vi "center_particle.vi"(0 "input_xyz":T4, 5 "tolerance":dbl=1e-06 format="%#_13g", 7 "max_iterations":i32=10, 9 "parameters_xy-scan":T2={"image_size_xy_um"=1.0, "frame_size_xy_px"=10, "dwell_time_ms"=1.0} {"dwell_time_ms" format="%#_13g"; "image_size_xy_um" format="%#_13g"}, 11 "parameters_z-scan":T1={"dwell_time_ms"=10.0, "q_steps"=10, "span_um"=1.0, "refocus"=TRUE} {"dwell_time_ms" format="%#_13g"}, 12 "autocorrect":bool=TRUE) -> (4 "output_xyz":T3, 6 "mini_scan":dbl[][](array[numeric]), 8 "timestamp":timestamp, 15 "particle_lost":bool)   [LabVIEW 2018]
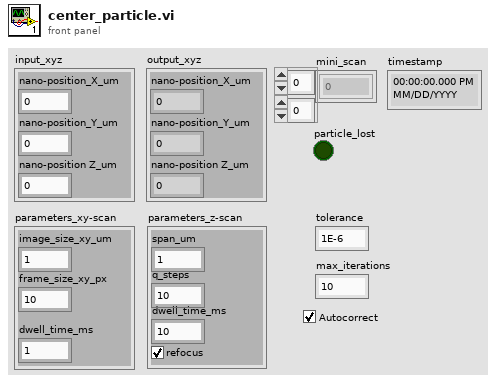
[diagram p1: front panel]
types:
  T1 = cluster{"dwell_time_ms":dbl, "q_steps":u32, "span_um":dbl, "refocus":bool}
  T2 = cluster{"image_size_xy_um":dbl, "frame_size_xy_px":u32, "dwell_time_ms":dbl}
  T3 = cluster{"nano-position_X_um":sgl, "nano-position_Y_um":sgl, "nano-position Z_um":sgl}
  T4 = cluster{"nano-position_X_um":dbl, "nano-position_Y_um":dbl, "nano-position Z_um":dbl}
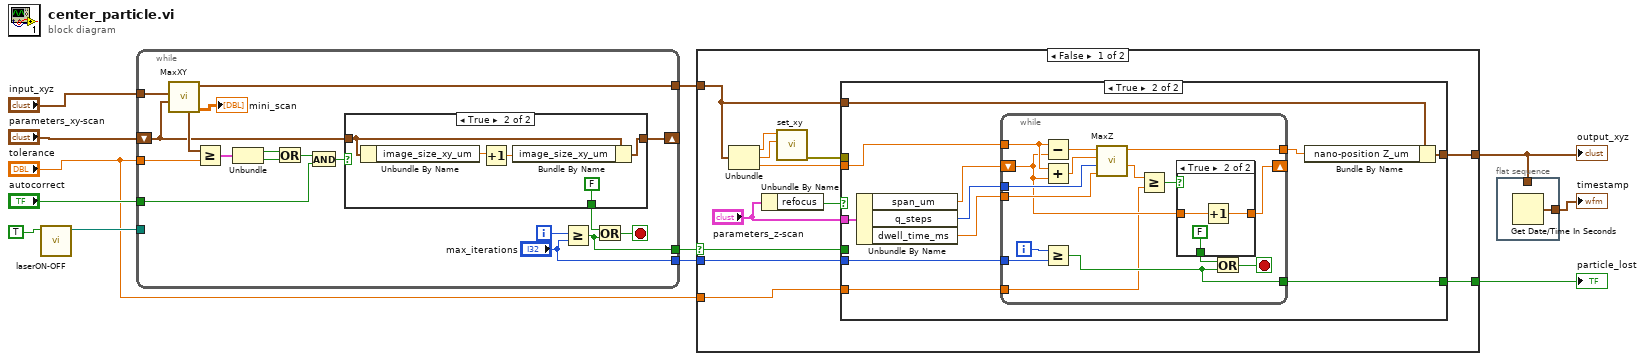
[diagram p0: block diagram]
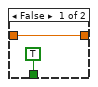
[diagram p3: hidden frame]
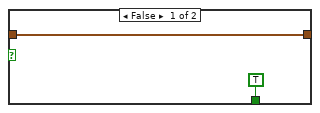
[diagram p5: hidden frame]
diagram:
  n1 = call "laserON-OFF.vi"("ON-OFF"=TRUE) -> ("path out"=w8:path)  [unwired: 10 in]
  n2 = while {
    tunnel: "input_xyz" -> [w30]
    tunnel: [w29] -> w11
    shift-right: [w22] -> _
    shift-left: "parameters_xy-scan" -> [w21]
    tunnel: "tolerance" -> [w16]
    tunnel: "autocorrect" -> [w15]
    tunnel: w8 -> [_]
    tunnel: [w14] -> w7
    tunnel: ["max_iterations"] -> w6
    i -> [w23]
    stop <- w20 stop-if-true
    n3 = call "MaxXY.vi"("input_xyz_um"=w30, "parameters_xy_scan"=w21) -> ("mse"=w27:cluster{"mse_y":dbl, "mse_x":dbl}, "output_xyz_um"=w29:T3, "image"=→"mini_scan":dbl[][])  [unwired: 4 in, 2 out]
    n4 = Greater Or Equal?(x=w27, y=w16) -> (x >= y?=w26:cluster{"mse_y":bool, "mse_x":bool})
    n5 = Unbundle(w26) -> ("mse_y"=w25:bool, "mse_x"=w24:bool)
    n6 = Or(x=w25, y=w24) -> (x .or. y?=w18:bool)
    n7 = And(x=w18, y=w15) -> (x .and. y?=w17:bool)
    n8 = case shown="True" w17 {
      tunnel: [w32 w33] -> w22
      tunnel: w21 -> [w32 w35]
      tunnel: [TRUE FALSE] -> w19
      frame False {
      }
      frame True {
        n9 = Unbundle By Name(w35) -> ("image_size_xy_um"=w36:dbl)
        n10 = Increment(x=w36) -> (x+1=w34:dbl)
        n11 = Bundle By Name(cluster=w35, "image_size_xy_um"=w34) -> (w33:T2)
      }
    }
    n12 = Greater Or Equal?(x=w23, y="max_iterations") -> (x >= y?=w14:bool)
    n13 = Or(x=w19, y=w14) -> (x .or. y?=w20:bool)
  }
  n14 = case shown="False" w7 {
    selector: w7 -> [w39 w84]
    tunnel: w11 -> [w43 w85]
    tunnel: w6 -> [w42 _]
    tunnel: [w41 w85] -> w2
    tunnel: [w40 w84] -> w3
    tunnel: "tolerance" -> [w38 _]
    frame False {
      n15 = Unbundle(w43) -> ("nano-position_X_um"=w45:sgl, "nano-position_Y_um"=w46:sgl, "nano-position Z_um"=w47:sgl)
      n16 = Unbundle By Name("parameters_z-scan") -> ("refocus"=w49:bool)
      n17 = call "set_xy.vi"("y_value_um"=w46, "x_value_um"=w45) -> ("error out"=w44:errorcluster)  [unwired: 9 in]
      n18 = case shown="True" w49 {
        tunnel: "parameters_z-scan" -> [_ w62]
        tunnel: [w51 w61] -> w41
        tunnel: w47 -> [_ w59]
        tunnel: w44 -> [_ _]
        tunnel: w43 -> [w51 w60]
        tunnel: w42 -> [_ w56]
        tunnel: [w50 w53] -> w40
        tunnel: w39 -> [w50 _]
        tunnel: w38 -> [_ w52]
        frame False {
        }
        frame True {
          n19 = Unbundle By Name(w62) -> ("span_um"=w58:dbl, "q_steps"=w57:u32, "dwell_time_ms"=w55:dbl)
          n20 = while {
            tunnel: w59 -> [w76]
            tunnel: w57 -> [w75]
            tunnel: w55 -> [w74]
            shift-right: [w69] -> _
            shift-left: w58 -> [w70]
            tunnel: w56 -> [w65]
            tunnel: [w71] -> w54
            tunnel: [w64] -> w53
            tunnel: w52 -> [w63]
            i -> [w66]
            stop <- w67 stop-if-true
            n21 = Subtract(x=w76, y=w70) -> (x-y=w78:dbl)
            n22 = Add(x=w76, y=w70) -> (x+y=w77:dbl)
            n23 = Greater Or Equal?(x=w66, y=w65) -> (x >= y?=w64:bool)
            n24 = call "MaxZ.vi"("dwell_time_ms"=w74, "q_steps"=w75, "z_end_um"=w77, "z_start_um"=w78) -> ("mse"=w73:dbl, "z_focus_um"=w71:dbl)  [unwired: 5 in, 1 out]
            n25 = Greater Or Equal?(x=w73, y=w63) -> (x >= y?=w72:bool)
            n26 = case shown="True" w72 {
              tunnel: w70 -> [w80 w83]
              tunnel: [w80 w82] -> w69
              tunnel: [TRUE FALSE] -> w68
              frame False {
              }
              frame True {
                n27 = Increment(x=w83) -> (x+1=w82:dbl)
              }
            }
            n28 = Or(x=w68, y=w64) -> (x .or. y?=w67:bool)
          }
          n29 = Bundle By Name(cluster=w60, "nano-position Z_um"=w54) -> (w61:T3)
        }
      }
    }
    frame True {
      # "Particle lost in MaxXY"
    }
  }
  "output_xyz" <- w2
  "particle_lost" <- w3
  n30 = flat-sequence {
    tunnel: [w86] -> w4
    tunnel: w2 -> [_]
    frame #0 {
      n31 = Get Date/Time In Seconds() -> (seconds since 1Jan1904=w86:timestamp)
    }
  }
  "timestamp" <- w4
